vi "NewEntry_DB.vi"(8 "error in (no error)":errorcluster, 11 "LotData in":refnum<class "LotData.lvclass">) -> (0 "error out":errorcluster, 2 "NewWaferEntry":string, 3 "LotData out":refnum<class "LotData.lvclass">)   [LabVIEW 2012, in "LotData.lvclass"]
uses:
  LotData.lvclass
  LotData.lvclass/LotData.ctl
  <vilib>/addons/database/Auxilliary.llb/DB Tools Parameter Info.ctl
  <vilib>/addons/database/Auxilliary.llb/DB Tools DataTypes.ctl
  <vilib>/addons/database/Auxilliary.llb/DB Tools Parameter Dir.ctl
  Controls/ProbeStationId.vi
  <vilib>/addons/database/Connection.llb/DB Tools Open Connec (Path).vi
  <vilib>/addons/database/Command.llb/Cmd Set Parameter Value (C).vi
  <vilib>/addons/database/Command.llb/Cmd Execute.vi
  <vilib>/addons/database/Recordset.llb/Rec Destroy - Command.vi
  <vilib>/addons/database/Command.llb/Cmd Delete.vi
  <vilib>/addons/database/NI_Database_API.lvlib
panel:
  out "Pocket":string
  out "Run Number":string
  out "System":string
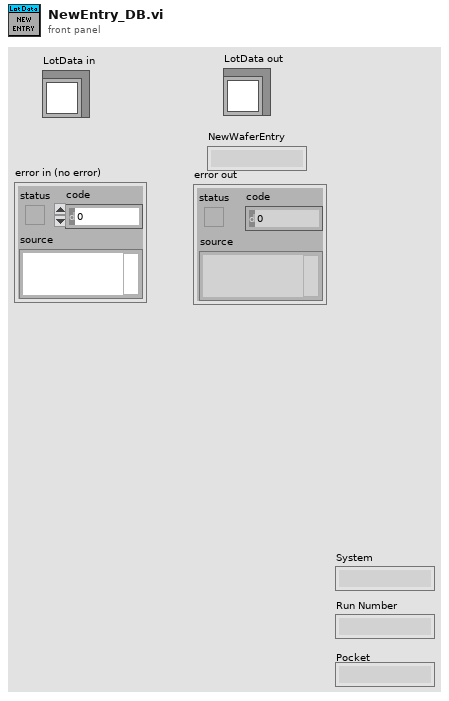
[diagram p1: front panel]
types:
  T1 = typedef "NI_Database_API.lvlib/DB Tools Parameter Info.ctl" = cluster{"parameter name":string, "type":T2, "direction":T3, "value":variant}
  T2 = typedef "NI_Database_API.lvlib/DB Tools DataTypes.ctl" = enum16{"String", "Long (I32)", "Single (SGL)", "Double (DBL)", "Date/Time", "Binary"}
  T3 = typedef "NI_Database_API.lvlib/DB Tools Parameter Dir.ctl" = enum32{"Input", "Output", "Input/Output", "Return Value"}
  T4 = typedef "NI_Database_API.lvlib/Conn ObjectReference.ctl" = refnum<k1>
  T5 = typedef "NI_Database_API.lvlib/Cmd ObjectReference.ctl" = refnum<k1>
  T6 = typedef "NI_Database_API.lvlib/Cmd-Rec Object Reference.ctl" = refnum<k1>
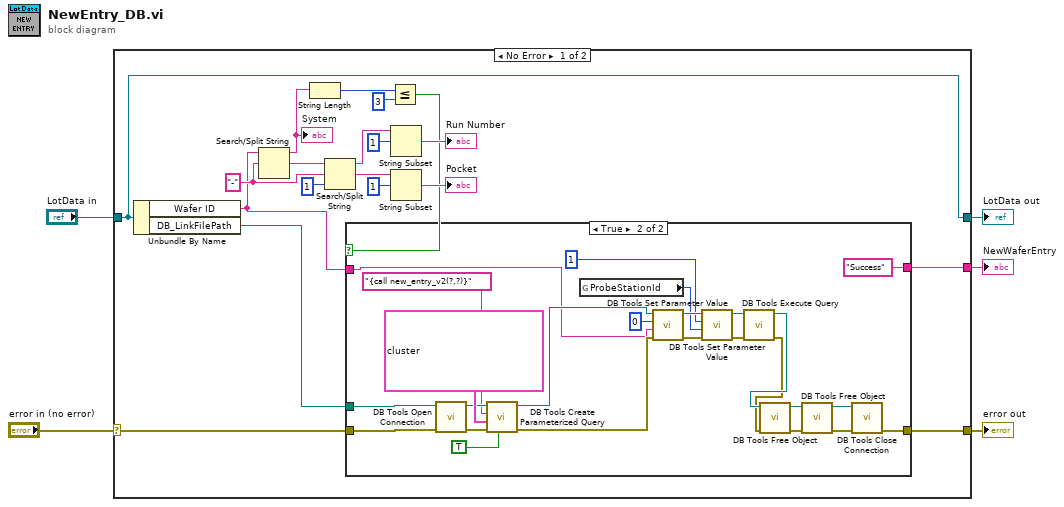
[diagram p0: block diagram]
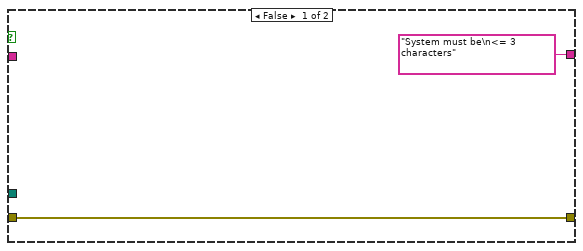
[diagram p2: hidden frame]
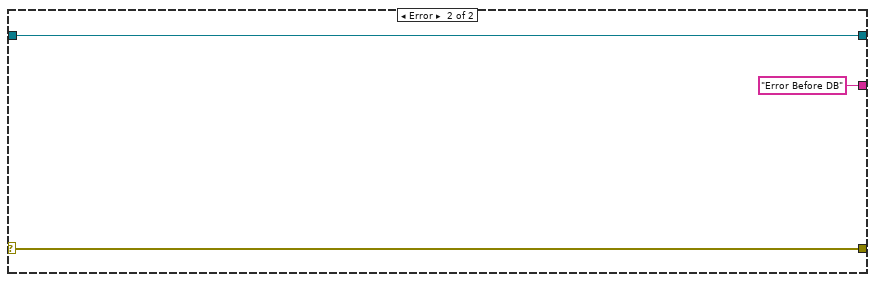
[diagram p3: hidden frame]
diagram:
  n1 = case shown="No Error" "error in (no error)" {
    selector: "error in (no error)" -> [w7 w54]
    tunnel: [w9 w54] -> w2
    tunnel: [w24 w53] -> w3
    tunnel: "LotData in" -> [w24 w53]
    tunnel: [w8 "Error Before DB" ("NewWaferEntry")] -> w1
    frame No Error {
      w22 = "-" ("search string/char (-)")
      n2 = Unbundle By Name(w24) -> ("Wafer ID"=w10:string, "DB_LinkFilePath"=w6:path)
      n3 = Search/Split String(string=w10, search string/char (-)=w22) -> (substring before match=w14:string, match + rest of string=w23:string)  [unwired: 1 in, 1 out]
      "System" <- w14
      n4 = String Length(string=w14) -> (length=w13:i32)
      n5 = Search/Split String(string=w23, search string/char (-)=w22, offset (0)=1) -> (substring before match=w17:string, match + rest of string=w20:string)  [unwired: 1 out]
      n6 = Less Or Equal?(x=w13, y=3) -> (x <= y?=w11:bool)
      n7 = case shown="True" w11 {
        tunnel: w10 -> [_ w29]
        tunnel: [w26 w43] -> w9
        tunnel: w7 -> [w26 w38]
        tunnel: ["System must be\n<= 3 characters" "Success"] -> w8
        tunnel: w6 -> [_ w36]
        frame False {
        }
        frame True {
          n8 = call-poly <vilib>:"DB Tools Open Connection.vi"("error in (no error)"=w38, "connection information"=w36) -> ("error out"=w48:errorcluster, "connection reference"=w49:T4)  [unwired: 6 in]
          n9 = call <vilib>:"DB Tools Create Parameterized Query.vi"("stored procedure? (F)"=TRUE, "error in (no error)"=w48, "parameters"=T1[] [{"parameter name"="wafer", "type"=enum."String", "direction"=enum."Input", "value"=variant}, {"parameter name"="stationId", "type"=enum."Long (I32)", "direction"=enum."Input", "value"=variant}], "SQL query"="{call new_entry_v2(?,?)}", "connection reference"=w49) -> ("error out"=w46:errorcluster, "command reference"=w45:T5)  [unwired: 2 in, 1 out]
          n10 = global read "ProbeStationId.vi" "ProbeStationId"() -> (w27:i32)
          n11 = call-poly <vilib>:"DB Tools Set Parameter Value.vi"("error in (no error)"=w46, "value"=w29, "parameter index"=0, "command reference"=w45) -> ("error out"=w32:errorcluster, "command reference out"=w33:T5)  [unwired: 4 in]
          n12 = call-poly <vilib>:"DB Tools Set Parameter Value.vi"("error in (no error)"=w32, "value"=w27, "parameter index"=1, "command reference"=w33) -> ("error out"=w31:errorcluster, "command reference out"=w30:T5)  [unwired: 4 in]
          n13 = call-poly <vilib>:"DB Tools Execute Query.vi"("error in (no error)"=w31, "command reference"=w30) -> ("error out"=w41:errorcluster, "command-recordset reference"=w42:T6)  [unwired: 6 in]
          n14 = call-poly <vilib>:"DB Tools Free Object.vi"("error in (no error)"=w41, "command-recordset reference"=w42) -> ("error out"=w44:errorcluster, "command reference"=w34:T5)  [unwired: 8 in]
          n15 = call-poly <vilib>:"DB Tools Free Object.vi"("error in (no error)"=w44, "command reference"=w34) -> ("error out"=w39:errorcluster, "connection reference"=w40:T4)  [unwired: 8 in]
          n16 = call <vilib>:"DB Tools Close Connection.vi"("error in (no error)"=w39, "connection reference"=w40) -> ("error out"=w43:errorcluster)  [unwired: 5 in]
        }
      }
      n17 = String Subset(string=w17, offset (0)=1) -> (substring=→"Run Number":string)  [unwired: 1 in]
      n18 = String Subset(string=w20, offset (0)=1) -> (substring=→"Pocket":string)  [unwired: 1 in]
    }
    frame Error {
    }
  }
  "error out" <- w2
  "LotData out" <- w3
  "NewWaferEntry" <- w1
